vi "ComboBoxFindValue(SubVI).vi"(1 "String":string, 2 "Strings and Values":cluster{"String":string, "Value":string}[](array[cluster])) -> (0 "Value":dbl)   [LabVIEW 2018]
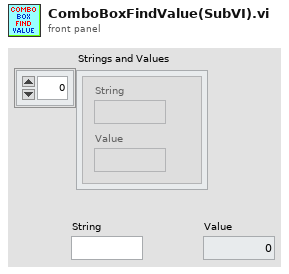
[diagram p1: front panel]
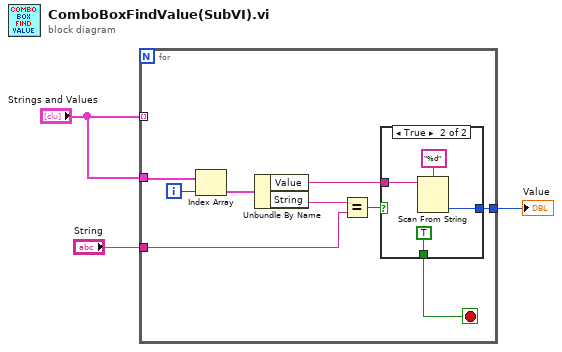
[diagram p0: block diagram]
diagram:
  n1 = for {
    tunnel: "Strings and Values" -> [_] mode=indexing
    tunnel: "Strings and Values" -> [w12]
    tunnel: "String" -> [w8]
    tunnel: [w5] -> w1
    i -> [w11]
    stop <- w4 stop-if-true
    n2 = Index Array(array=w12, index=w11) -> (element=w10:cluster{"String":string, "Value":string})
    n3 = Unbundle By Name(w10) -> ("Value"=w6:string, "String"=w9:string)
    n4 = Equal?(x=w9, y=w8) -> (x = y?=w7:bool)
    n5 = case shown="True" w7 {
      tunnel: w6 -> [_ w16]
      tunnel: [_ w15] -> w5
      tunnel: [_ TRUE] -> w4
      frame False {
      }
      frame True {
        n6 = Scan From String(format string="%d", input string=w16) -> (output 1=w15:i32)  [unwired: 3 in, 3 out]
      }
    }
  }
  "Value" <- w1
